vi "QSend.vi"(8 "error in (no error)":errorcluster, 11 "Command":string) -> (0 "error out":errorcluster)   [LabVIEW 2020, in "ErrorHandler.lvlib"]
doc: "Sends a message to the owning module"
uses:
  ErrorHandler.lvlib
  Controls/QMessage.ctl
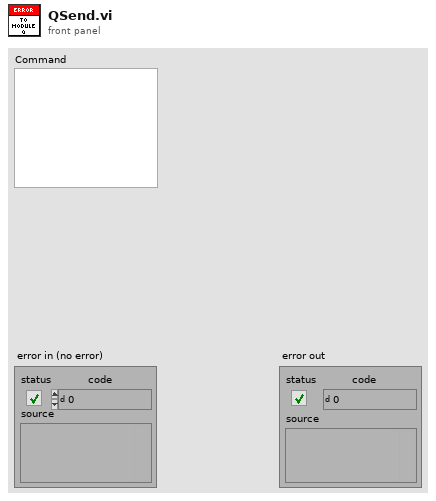
[diagram p1: front panel]
types:
  T1 = typedef "ErrorHandler.lvlib/QMessage.ctl" = cluster{"Message":string, "Data":errorcluster}
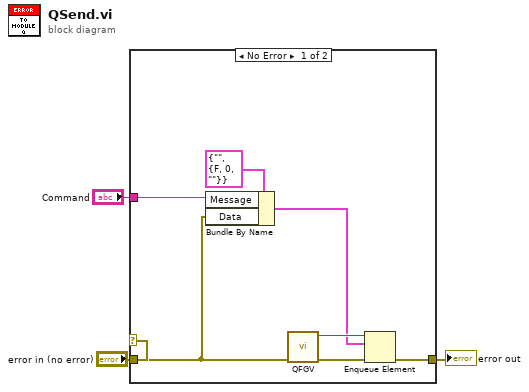
[diagram p0: block diagram]
diagram:
  n1 = case shown="No Error" "error in (no error)" {
    tunnel: [w7 w11] -> w3
    tunnel: "error in (no error)" -> [w4 w11]
    tunnel: "Command" -> [w5 _]
    frame No Error {
      n2 = Bundle By Name(cluster=T1 {"Message"="", "Data"={"status"=FALSE, "code"=0, "source"=""}}, "Message"=w5, "Data"=w4) -> (w6:T1)
      n3 = call "QFGV.vi"("error in (no error)"=w4) -> ("error out"=w10:errorcluster, "ModuleQ"=w8:refnum<queue>)  [unwired: 9 in]
      n4 = Enqueue Element(queue=w8, element=w6, error in (no error)=w10) -> (error out=w7:errorcluster)  [unwired: 1 in, 2 out]
    }
    frame Error {
    }
  }
  "error out" <- w3
